vi "Queue FGV.vi"(8 "error in (no error)":errorcluster, 11 "Queue FGV  Action":T1) -> (0 "error out":errorcluster, 3 "queue out":refnum<queue>)   [LabVIEW 2020, in "User Console.lvlib"]
doc: "For named purposes"
uses:
  User Console.lvlib
  Private Control/Queue FGV Action.ctl
  Private Control/Queue Element.ctl
  Private Control/Module Action.ctl
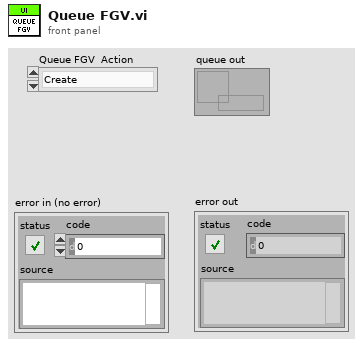
[diagram p1: front panel]
types:
  T1 = typedef "User Console.lvlib/Queue FGV Action.ctl" = enum16{"Create", "Get", "Release"}
  T2 = typedef "User Console.lvlib/Queue Element.ctl" = cluster{"Module Action":T3, "Data":variant}
  T3 = typedef "User Console.lvlib/Module Action.ctl" = enum16{"Init", "Error", "Exit"}
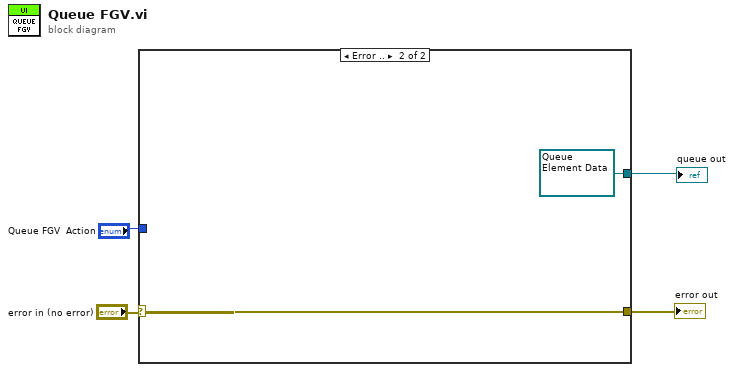
[diagram p0: block diagram]
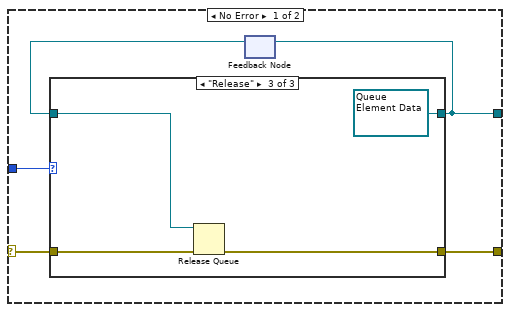
[diagram p2: hidden frame]
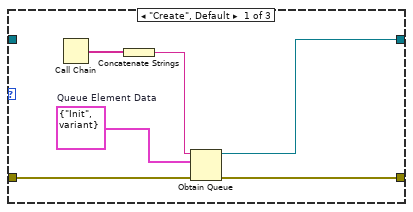
[diagram p3: hidden frame]
diagram:
  n1 = case shown="Error .." "error in (no error)" {
    selector: "error in (no error)" -> [w8 w23]
    tunnel: [w7 w23] -> w3
    tunnel: "Queue FGV  Action" -> [w9 _]
    tunnel: [w5 refnum<queue> refnum ("queue out")] -> w1
    frame No Error {
      n2 = feedback #1() -> (w6:refnum<queue>)  [unwired: 1 in]
      n3 = case shown="\"Release\"" w9 {
        tunnel: w8 -> [w12 w16 w20]
        tunnel: [w11 w16 w19] -> w7
        tunnel: [w10 w17 refnum<queue> refnum ("queue out")] -> w5
        tunnel: w6 -> [_ w17 w21]
        frame "Create", Default {
          w13 = T2 {"Module Action"=enum."Init", "Data"=variant}  # Queue Element Data
          n4 = Call Chain() -> (call chain=w15:string[])
          n5 = Concatenate Strings(w15) -> (w14:string)
          n6 = Obtain Queue(name (unnamed)=w14, element data type=w13, error in (no error)=w12) -> (queue out=w10:refnum<queue>, error out=w11:errorcluster)  [unwired: 2 in, 1 out]
        }
        frame "Get" {
        }
        frame "Release" {
          n7 = Release Queue(queue=w21, error in (no error)=w20) -> (error out=w19:errorcluster)  [unwired: 1 in, 2 out]
        }
      }
      n8 = feedback-in #1(w5) -> ()
    }
    frame Error {
    }
  }
  "error out" <- w3
  "queue out" <- w1
